vi "MHD_reconstruction_Eng.vi"(1 "Number of harmonics":u8, 3 "Modulation amplitude (mT)":sgl, 4 "X":csg[](array[numeric]), 5 "Scan width":sgl, 7 "Number of points / scan":u32, 8 "Input spectra":csg[](array[numeric])) -> (0 "Fn":cdb[](array[numeric]), 2 "Dn":cdb[][](array[numeric]), 6 "Harmonics spectra":dbl[][](array[numeric]))   [LabVIEW 2020]
uses:
  <vilib>/Analysis/2dsp.llb/Complex FFT.vi
  <vilib>/Analysis/2dsp.llb/Inverse Real FFT.vi
  <vilib>/gmath/NI_Gmath.lvlib
  <vilib>/Analysis/NI_AALPro.lvlib
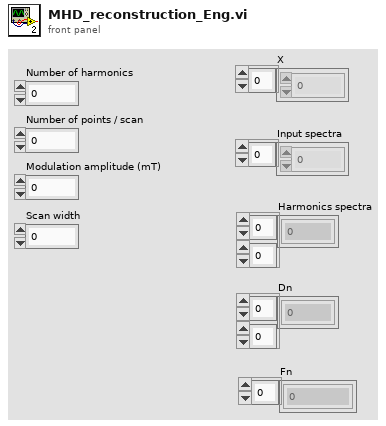
[diagram p1: front panel]
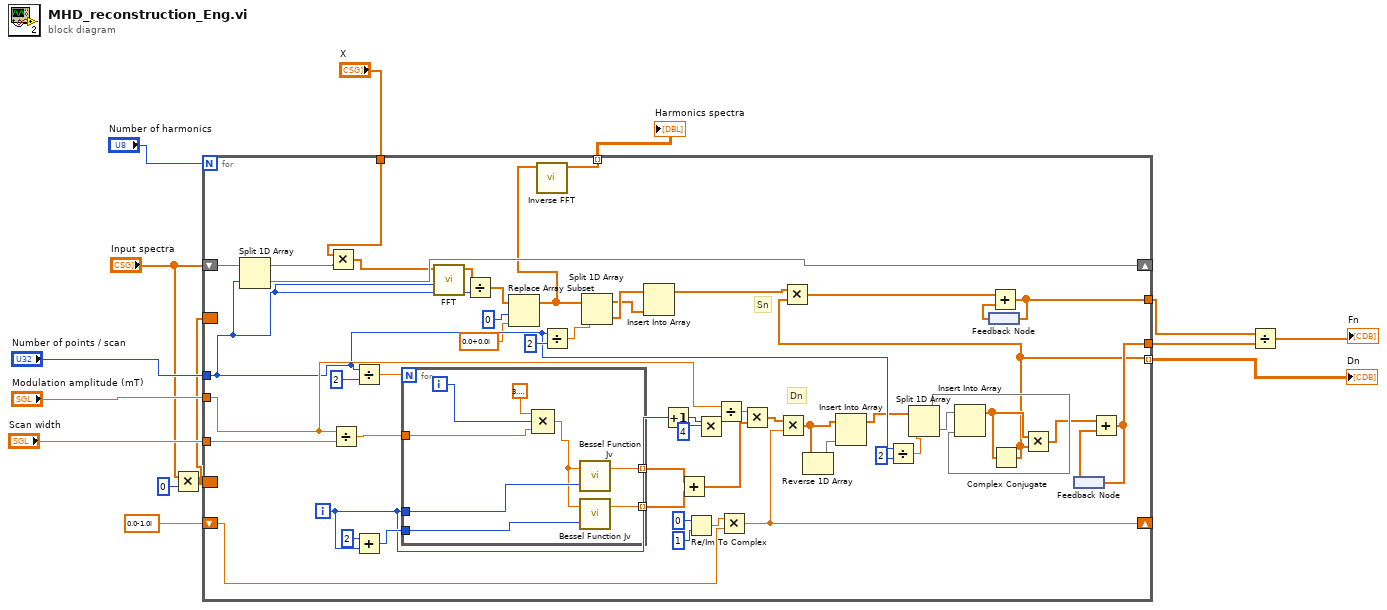
[diagram p0: block diagram]
diagram:
  n1 = Multiply(x="Input spectra", y=u8 0) -> (x*y=w4:csg[])
  n2 = for {
    N: "Number of harmonics" -> [_]
    tunnel: "Modulation amplitude (mT)" -> [w43]
    tunnel: "Number of points / scan" -> [w31]
    shift-right: [w57] -> _
    shift-left: csg 0.0-1.0i -> [w55]
    tunnel: "Scan width" -> [w53]
    shift-right: [w58] -> _
    shift-left: "Input spectra" -> [w59]
    tunnel: [w37] -> w9
    tunnel: [w35] -> w8
    border: w4 -> [_]
    border: w4 -> [_]
    tunnel: [w20] -> w3 mode=indexing
    tunnel: [w18] -> w2 mode=indexing
    tunnel: "X" -> [w16]
    i -> [w46]
    # "Sn"
    # "Dn"
    n3 = Split 1D Array(array=w59, index=w31) -> (first subarray=w17:csg[], second subarray=w58:csg[])
    n4 = Multiply(x=w16, y=w17) -> (x*y=w15:csg[])
    n5 = Divide(x=w43, y=w53) -> (x/y=w52:sgl)
    n6 = Divide(x=w31, y=u8 2) -> (x/y=w32:dbl)
    n7 = Add(x=u8 2, y=w46) -> (x+y=w49:i32)
    n8 = for {
      N: w32 -> [_]
      tunnel: [w75] -> w47 mode=indexing
      tunnel: [w70] -> w50 mode=indexing
      tunnel: w46 -> [w74]
      tunnel: w49 -> [w71]
      tunnel: w52 -> [w72]
      i -> [w68]
      n9 = Compound Arithmetic op=MULTIPLY(sgl 3.1415927, w68, w72) -> (w69:sgl)
      n10 = call <vilib>:"Bessel Function Jv.vi"("v"=w74, "x"=w69) -> ("Jv(x)"=w70:dbl)  [unwired: 1 in]
      n11 = call <vilib>:"Bessel Function Jv.vi"("v"=w71, "x"=w69) -> ("Jv(x)"=w75:dbl)  [unwired: 1 in]
    }
    n12 = call-poly <vilib>:"FFT.vi"("FFT size"=w31, "X"=w15) -> ("FFT {X}"=w42:cdb[])  [unwired: 8 in, 1 out]
    n13 = Divide(x=w42, y=w31) -> (x/y=w22:cdb[])
    n14 = Replace Array Subset(array=w22, new element=cdb 0.0+0.0i ("new element/subarray"), index=0) -> (w19:cdb[])
    n15 = call-poly <vilib>:"Inverse FFT.vi"("FFT {X}"=w19) -> ("X"=w20:dbl[])  [unwired: 9 in, 1 out]
    n16 = Divide(x=w31, y=u8 2) -> (x/y=w61:dbl)
    n17 = Split 1D Array(array=w19, index=w61) -> (first subarray=w62:cdb[], second subarray=w63:cdb[])
    n18 = Insert Into Array(array=w63, new element=w62) -> (w24:cdb[])  [unwired: 1 in]
    n19 = Increment(x=w46) -> (x+1=w64:i32)
    n20 = Add ("和")(x=w50, y=w47) -> (x+y=w51:dbl[])
    n21 = Re/Im To Complex(1:u8 1 ("y"), 2:u8 0 ("x")) -> (0:w56:cdb)
    n22 = Multiply(x=w64, y=u8 4) -> (x*y=w45:i32)
    n23 = Divide(x=w43, y=w45) -> (x/y=w44:sgl)
    n24 = Multiply(x=w56, y=w55) -> (x*y=w57:cdb)
    n25 = Multiply ("積")(x=w44, y=w51) -> (x*y=w48:dbl[])
    n26 = Multiply ("積")(x=w48, y=w57) -> (x*y=w29:cdb[])
    n27 = Reverse 1D Array(array=w29) -> (reversed array=w28:cdb[])
    n28 = Insert Into Array(array=w29, new element=w28) -> (w27:cdb[])  [unwired: 1 in]
    n29 = Divide(x=w31, y=u8 2) -> (x/y=w41:dbl)
    n30 = Split 1D Array(array=w27, index=w41) -> (first subarray=w39:cdb[], second subarray=w34:cdb[])
    n31 = Insert Into Array(array=w34, new element=w39) -> (w26:cdb[])  [unwired: 1 in]
    n32 = feedback #1() -> (w38:cdb[])
    n33 = Complex Conjugate ("複素共役")(1:w26) -> (0:w18:cdb[])
    n34 = Multiply(x=w24, y=w18) -> (x*y=w33:cdb[])
    n35 = Add(x=w33, y=w38) -> (x+y=w37:cdb[])
    n36 = feedback-in #1(w37) -> ()
    n37 = Multiply(x=w26, y=w18) -> (x*y=w25:cdb[])
    n38 = feedback #2() -> (w36:cdb[])
    n39 = Add(x=w25, y=w36) -> (x+y=w35:cdb[])
    n40 = feedback-in #2(w35) -> ()
  }
  "Harmonics spectra" <- w3
  "Dn" <- w2
  n41 = Divide(x=w9, y=w8) -> (x/y=→"Fn":cdb[])
